vi "hexStringToByteData.vi"(9 "数据输入":string, 10 "协议":u32(ring) items=["CAN", "CANFD"]) -> (0 "Array":u32[](array[numeric]), 1 "CANFD_data":T1, 2 "CAN_data":T2, 3 "字节数":u8)   [LabVIEW 2020, in "zlgcan.lvlib"]
uses:
  zlgcan.lvlib
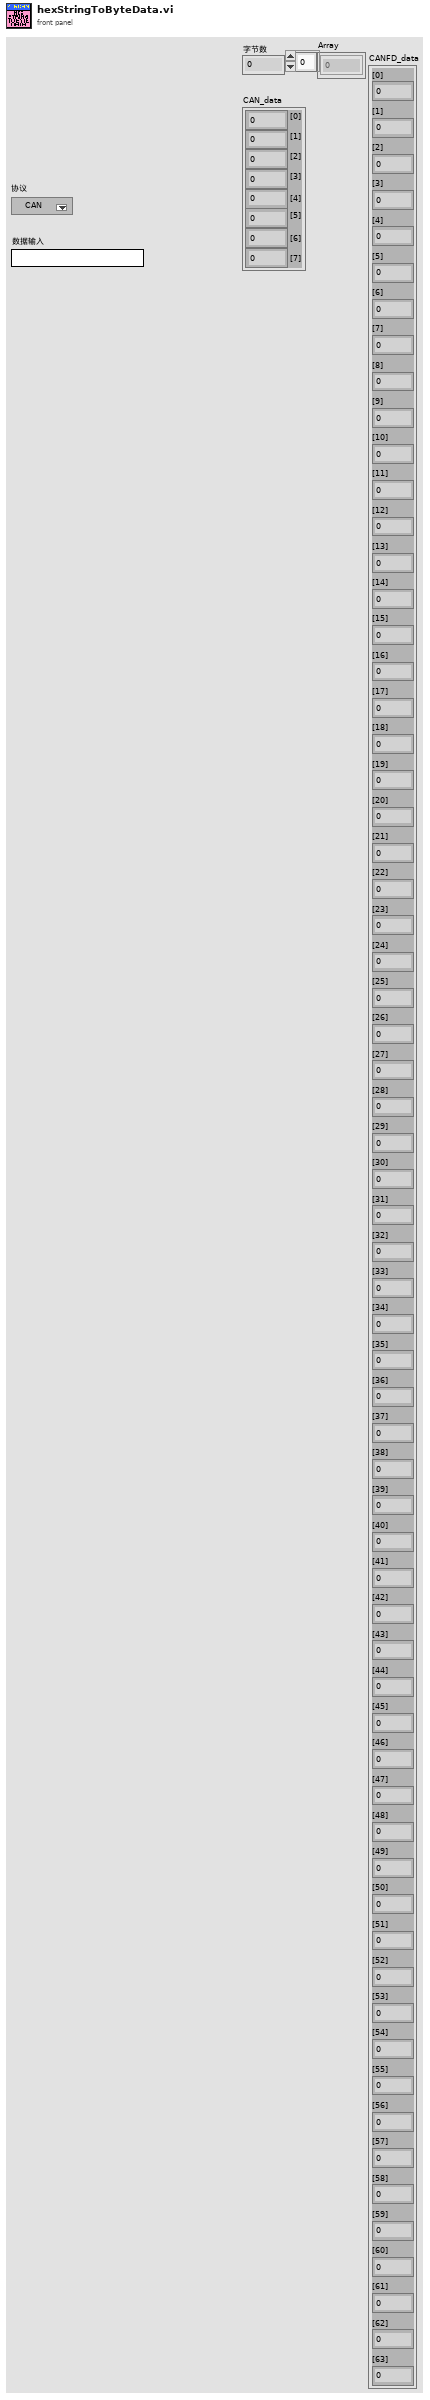
[diagram p1: front panel]
types:
  T1 = cluster{"[0]":u32, "[1]":u32, "[2]":u32, "[3]":u32, "[4]":u32, "[5]":u32, "[6]":u32, "[7]":u32, "[8]":u32, "[9]":u32, "[10]":u32, "[11]":u32, "[12]":u32, "[13]":u32, "[14]":u32, "[15]":u32, "[16]":u32, "[17]":u32, "[18]":u32, "[19]":u32, "[20]":u32, "[21]":u32, "[22]":u32, "[23]":u32, "[24]":u32, "[25]":u32, "[26]":u32, "[27]":u32, "[28]":u32, "[29]":u32, "[30]":u32, "[31]":u32, "[32]":u32, "[33]":u32, "[34]":u32, "[35]":u32, "[36]":u32, "[37]":u32, "[38]":u32, "[39]":u32, "[40]":u32, "[41]":u32, "[42]":u32, "[43]":u32, "[44]":u32, "[45]":u32, "[46]":u32, "[47]":u32, "[48]":u32, "[49]":u32, "[50]":u32, "[51]":u32, "[52]":u32, "[53]":u32, "[54]":u32, "[55]":u32, "[56]":u32, "[57]":u32, "[58]":u32, "[59]":u32, "[60]":u32, "[61]":u32, "[62]":u32, "[63]":u32}
  T2 = cluster{"[0]":u8, "[1]":u32, "[2]":u32, "[3]":u32, "[4]":u32, "[5]":u32, "[6]":u32, "[7]":u32}
  T3 = cluster{"[0]":u32, "[1]":u32, "[2]":u32, "[3]":u32, "[4]":u32, "[5]":u32, "[6]":u32, "[7]":u32}
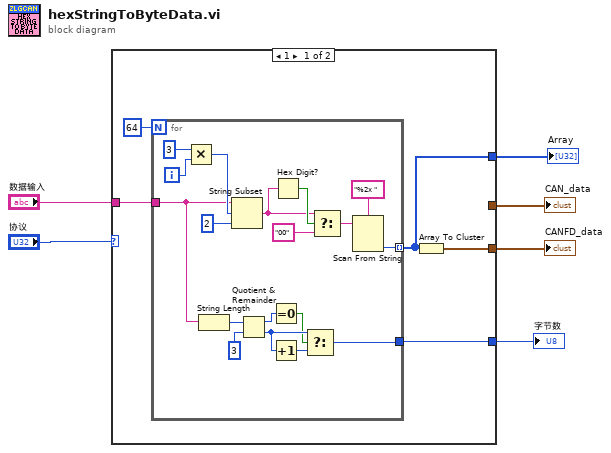
[diagram p0: block diagram]
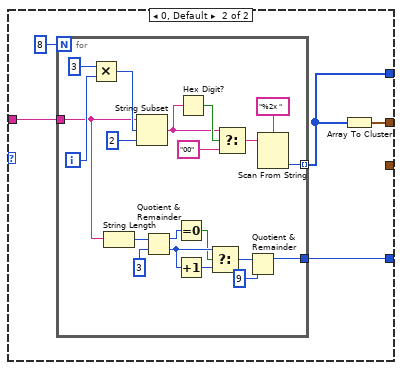
[diagram p2: hidden frame]
diagram:
  n1 = case shown="1" "协议" {
    tunnel: "数据输入" -> [w10 w34]
    tunnel: [w9 w32] -> w5
    tunnel: [_ w31] -> w3
    tunnel: [w8 _] -> w2
    tunnel: [w7 w30] -> w1
    frame 1 {
      n2 = for {
        N: 64 -> [_]
        tunnel: w10 -> [w14]
        tunnel: [w25] -> w7 mode=indexing
        tunnel: [w12] -> w9
        i -> [w20]
        n3 = Multiply(x=3, y=w20) -> (x*y=w28:i32)
        n4 = String Length(string=w14) -> (length=w19:i32)
        n5 = String Subset(string=w14, offset (0)=w28, length (rest)=2 ("length (rest)")) -> (substring=w22:string)
        n6 = Quotient & Remainder(x=w19, y=3) -> (x-y*floor(x/y)=w17:i32, floor(x/y)=w15:i32)
        n7 = Equal To 0?(x=w17) -> (x = 0?=w13:bool)
        n8 = Increment(x=w15) -> (x+1=w16:i32)
        n9 = Hex Digit?(1:w22) -> (0:w23:bool)
        n10 = Select(t=w15, s=w13, f=w16) -> (s? t:f=w12:i32)
        n11 = Select(t=w22, s=w23, f="00" ("t")) -> (s? t:f=w24:string)
        n12 = Scan From String(format string="%2x ", input string=w24) -> (output 1=w25:u32)  [unwired: 2 in, 4 out]
      }
      n13 = Array To Cluster(array=w7) -> (cluster=w8:T1)
    }
    frame 0, Default {
      n14 = for {
        N: 8 -> [_]
        tunnel: w34 -> [w37]
        tunnel: [w50] -> w30 mode=indexing
        tunnel: [w36] -> w32
        i -> [w45]
        n15 = Multiply(x=3, y=w45) -> (x*y=w53:i32)
        n16 = String Length(string=w37) -> (length=w44:i32)
        n17 = String Subset(string=w37, offset (0)=w53, length (rest)=2 ("length (rest)")) -> (substring=w47:string)
        n18 = Quotient & Remainder(x=w44, y=3) -> (x-y*floor(x/y)=w42:i32, floor(x/y)=w40:i32)
        n19 = Equal To 0?(x=w42) -> (x = 0?=w35:bool)
        n20 = Increment(x=w40) -> (x+1=w41:i32)
        n21 = Hex Digit?(1:w47) -> (0:w48:bool)
        n22 = Select(t=w40, s=w35, f=w41) -> (s? t:f=w39:i32)
        n23 = Select(t=w47, s=w48, f="00" ("t")) -> (s? t:f=w49:string)
        n24 = Quotient & Remainder(x=w39, y=9) -> (x-y*floor(x/y)=w36:i32)  [unwired: 1 out]
        n25 = Scan From String(format string="%2x ", input string=w49) -> (output 1=w50:u32)  [unwired: 2 in, 4 out]
      }
      n26 = Array To Cluster(array=w30) -> (cluster=w31:T3)
    }
  }
  "字节数" <- w5
  "CAN_data" <- w3
  "CANFD_data" <- w2
  "Array" <- w1
